vi "PoC writer Eth.vi"() -> ()   [LabVIEW 2022 SP3]
uses:
  JLR/emea-tra-JLR-Synchronization-PoC/PoC_LV2020/Data.ctl
  JLR/emea-tra-JLR-Synchronization-PoC/PoC_LV2020/States.ctl
  <vilib>/xnet/xnet.llb/XNET Frame Ethernet.ctl
  <vilib>/xnet/xnet.llb/XNET Frame Type Ethernet.ctl
  Program Files/National Instruments/LabVIEW 2022/examples/nixnet/projects/NI-XNET Ethernet/subVI/Ethernet/Controls/Ethernet Header.ctl
  Program Files/National Instruments/LabVIEW 2022/examples/nixnet/projects/NI-XNET Ethernet/subVI/Ethernet/Controls/VLAN Tag.ctl
  87a1c0d7-935f-47c0-8fc5-bd666b1ac1f8.vi
  <vilib>/xnet/xnet.llb/XNET Read (State Time Current).vi
  <instrlib>/niSync/niSync.llb/niSync Initialize (Default).vi
  <vilib>/xnet/xnet.llb/XNET Create Session (Frame Output Stream).vi
  <vilib>/xnet/xnet.llb/XNET Write (Frame Ethernet).vi
  <vilib>/xnet/xnet.llb/XNET Read (State Time Trigger).vi
  <resource>/objmgr/xnet.rc
  Program Files/National Instruments/LabVIEW 2022/examples/nixnet/projects/NI-XNET Ethernet/subVI/Ethernet.lvlib
panel:
  out "TimeStamps":timestamp[](array[timestamp]) format="%<%.6X\n%x>T"
  in  "terminal":tag="/Dev2/PFI0"
  in  "terminal 2":tag="/Dev2/PXI_Trig0"
  in  "resource name 2":tag="Dev2"
  in  "Start Time Delay (Seconds)":ext=1.0
  in  "Pulse Width (uS)":ext=1.0
  out "Pulse Start Time":timestamp format="%<%I:%M:%S%6u %p\n%x>T"
  in  "Send Trigger":bool
  out "Time Trigger Received":timestamp caption="network time trigger" format="%<%.6X\n%x>T"
  out "UTC Offset (s)":i32
  out "Port State":u32(ring)=3 items=["Disabled"=3, "Master"=6, "Passive"=7, "Slave"=9]
  out "Time Diff (Sync vs Xnet) (s)":dbl format="%#.6f"
  out "Adj Time Diff (Sync vs Xnet) (s)":dbl format="%#.6f"
  in  "payload 2":string="\u0000\u0001\u0002\u0003\u0004\u0005\u0006\u0007\b\t\n\u000b\f\r\u000e\u000f\u0010\u0011\u0012\u0013\u0014\u0015\u0016\u0017\u0018\u0019\u001a\u001b\u001c\u001d\u001e\u001f !\"#$%&'()*+,-./0123456789:;<=>?@ABCDEFGHIJKLMNOPQRSTUVWXYZ[\\]^_`abc"
  in  "destination MAC address":cluster{u8, u8, u8, u8, u8, u8}={255, 255, 255, 255, 255, 255} {"?" format="%.0x"; "?" format="%.0x"; "?" format="%.0x"; "?" format="%.0x"; "?" format="%.0x"; "?" format="%.0x"}
  in  "Has VLAN Tag":bool=TRUE
  in  "Ethertype":u16=34997 format="%.0x"
  in  "VID":u16=2
  in  "priority":u8=3
  in  "Write Frame":bool
  out "Frames sent":u32
  out "Time elapsed to set OS time (s)":dbl format="%#.6f"
  in  "gPtP master interface":refnum<k21>="ENET1"
  in  "NI Sync Resource Name":tag="Dev2"
  in  "Stop 2":bool
  out "Cluster":T1 {"OS time set at" format="%<%.6X\n%x>T"; "Time Trigger Received" format="%<%.6X\n%x>T"}
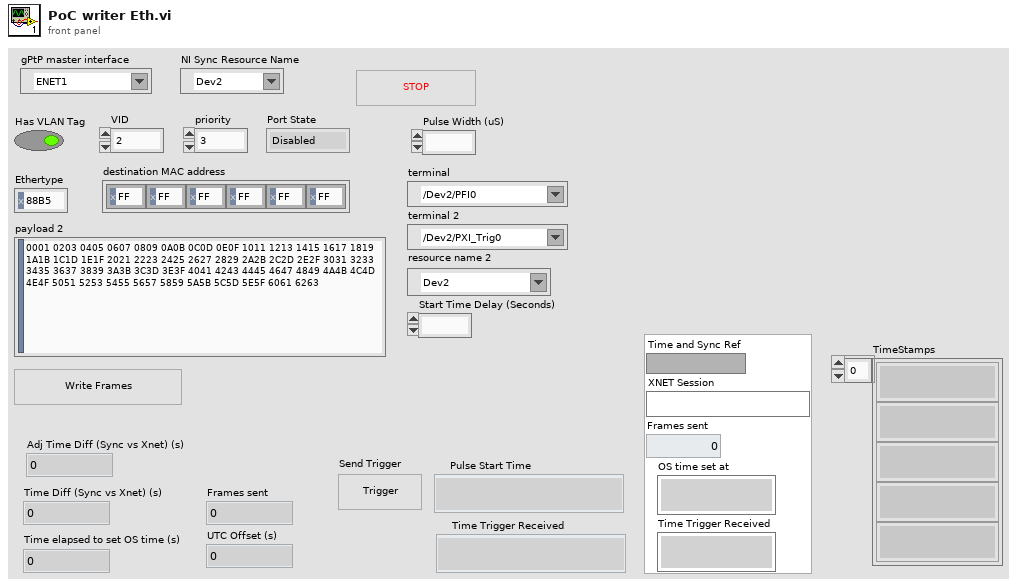
[diagram p1: front panel]
types:
  T1 = typedef "Data.ctl" = cluster{"Time and Sync Ref":refnum<k15>, "XNET Session":refnum<k21>, "Frames sent":u32, "OS time set at":timestamp, "Time Trigger Received":timestamp}
  T2 = enum16{"open", "open or create", "create or replace", "create", "open (read-only)"}
  T3 = typedef "States.ctl" = enum16{"Init 8523", "Init 6683", "Sync 8523", "PPS+Trigger", "Set Sync Time", "Init 8510", "Adjust XNET time", "Idle", "Error"}
  T4 = typedef "States.ctl" = enum16{"Init NI Sync", "Adjust XNET time", "Init XNET", "Update OS time", "Write XNET Frame", "Error", "Idle", "Read Trigger"}
  T5 = typedef "Ethernet.lvlib/VLAN Tag.ctl" = cluster{"TPID":u16, "priority":u8, "DEI":bool, "VID":u16}
  T6 = typedef "Ethernet.lvlib/Ethernet Header.ctl" = cluster{"destination MAC address":cluster{u8, u8, u8, u8, u8, u8}, "source MAC address":cluster{u8, u8, u8, u8, u8, u8}, "Has VLAN Tag":bool, "VLAN Tag":T5, "Ethertype":u16}
  T7 = typedef "XNET Frame Ethernet.ctl" = cluster{"local timestamp":timestamp, "network timestamp":timestamp, "frame data":u8[], "fcs":u32, "type":T8, "network synced?":bool, "receive?":bool, "transmit?":bool, "error?":bool}
  T8 = typedef "XNET Frame Type Ethernet.ctl" = u16
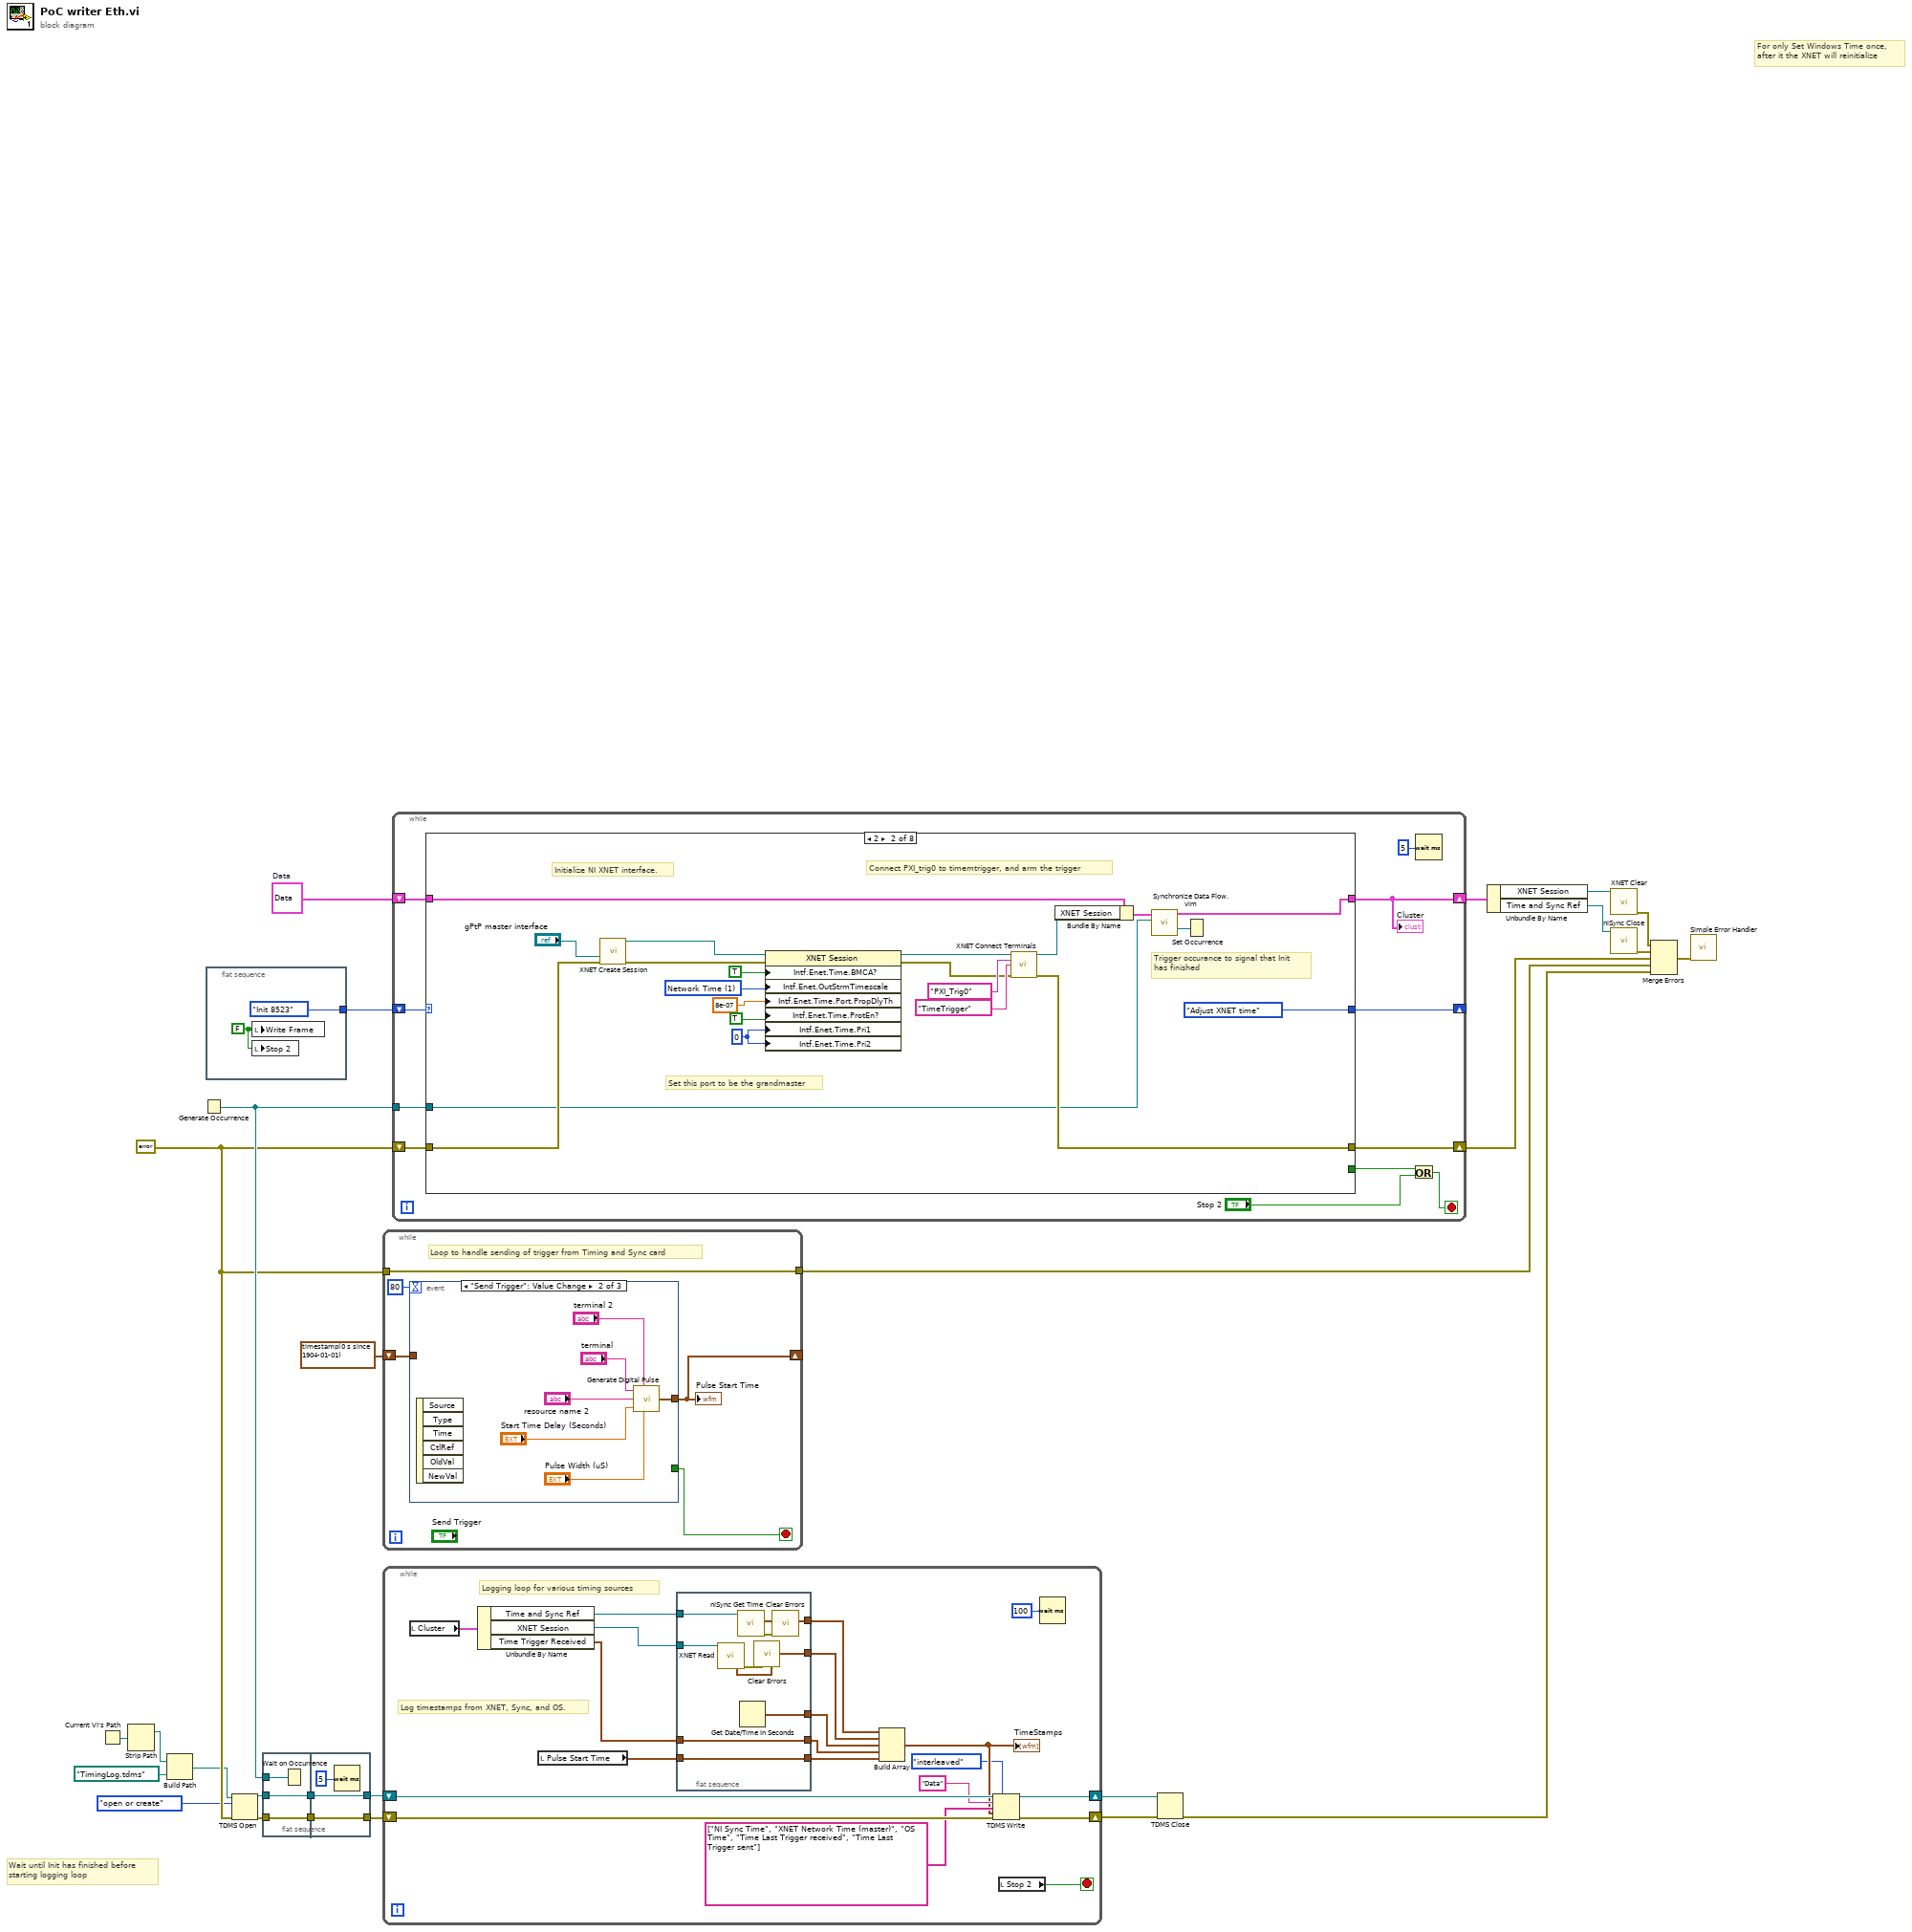
[diagram p0: block diagram]
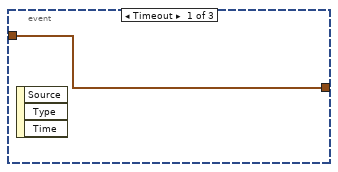
[diagram p2: hidden frame]
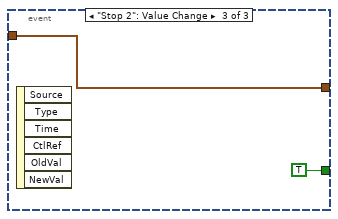
[diagram p3: hidden frame]
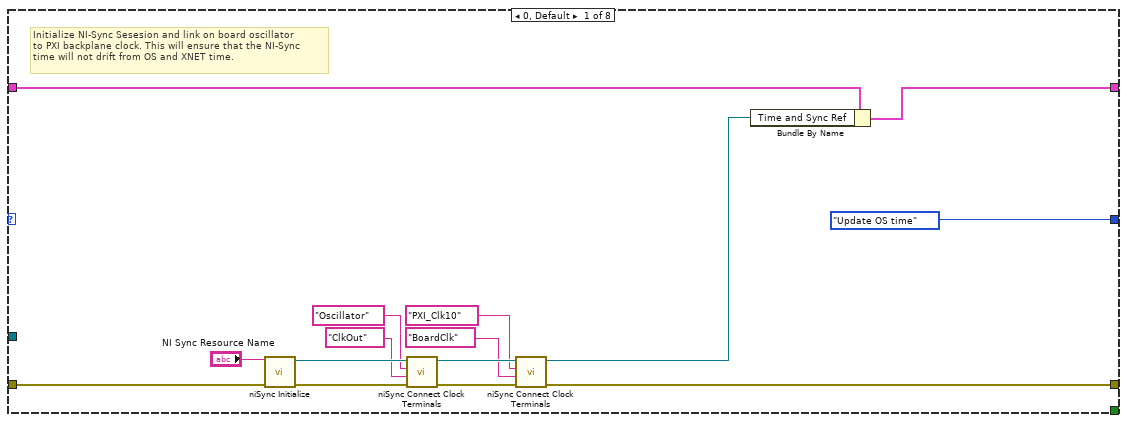
[diagram p4: hidden frame]
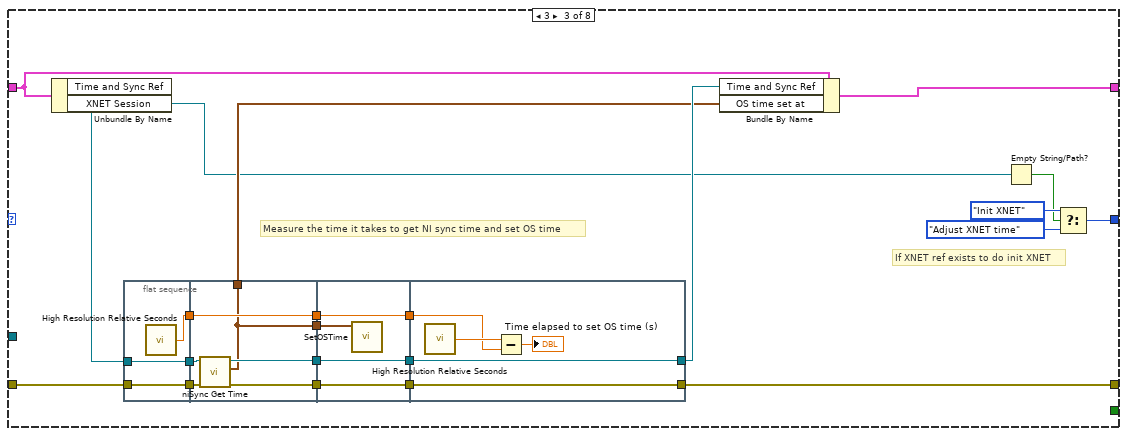
[diagram p5: hidden frame]
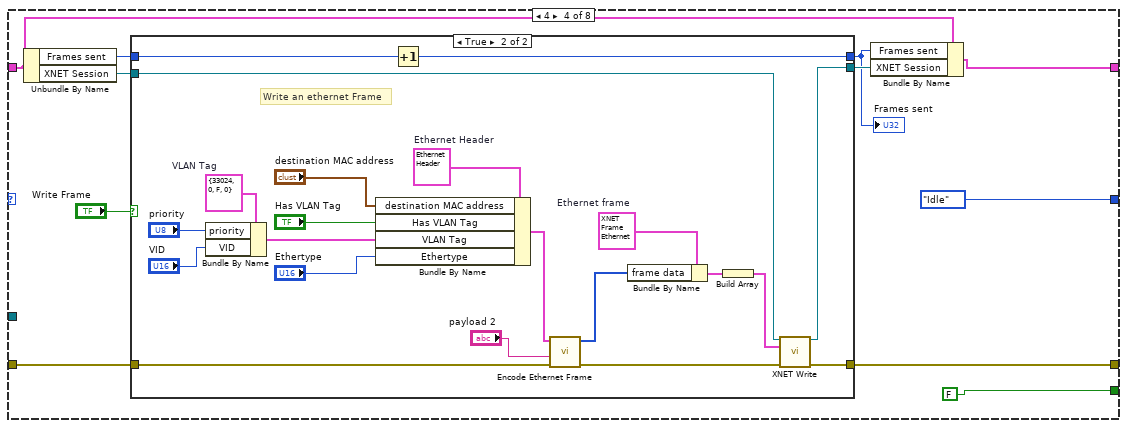
[diagram p6: hidden frame]
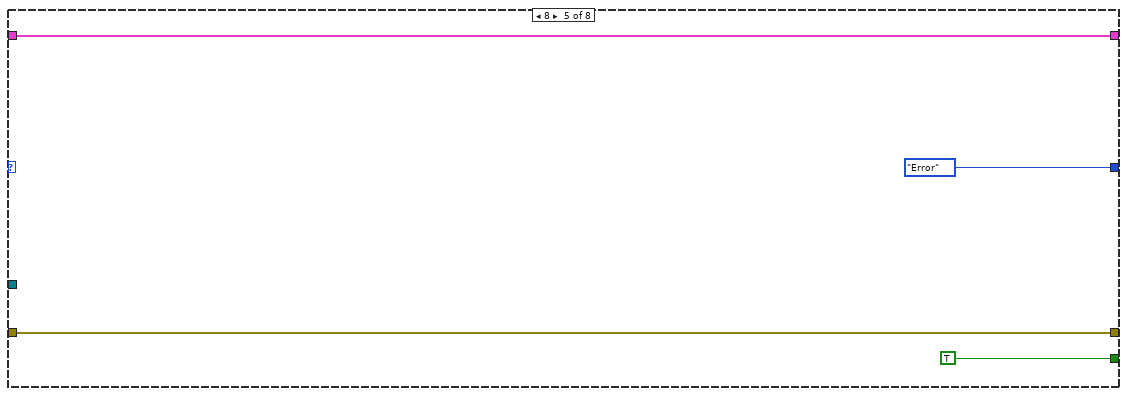
[diagram p8: hidden frame]
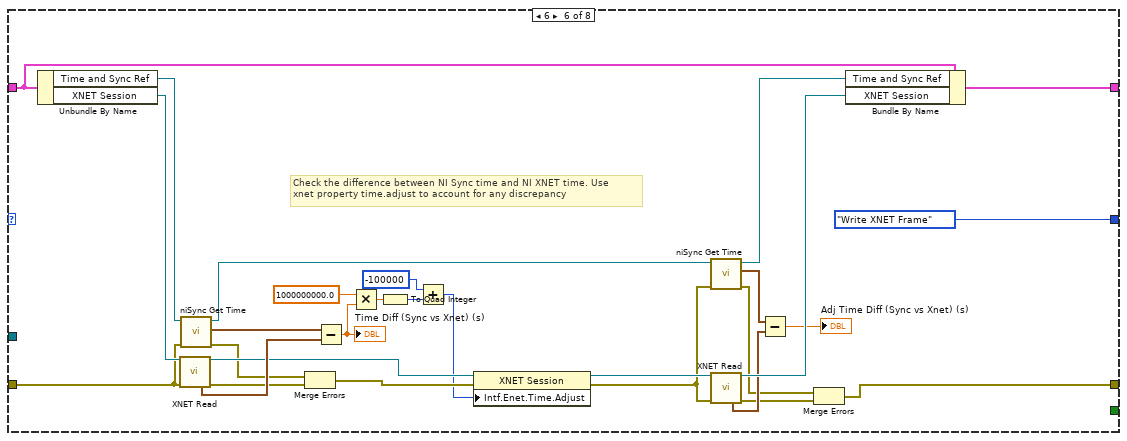
[diagram p9: hidden frame]
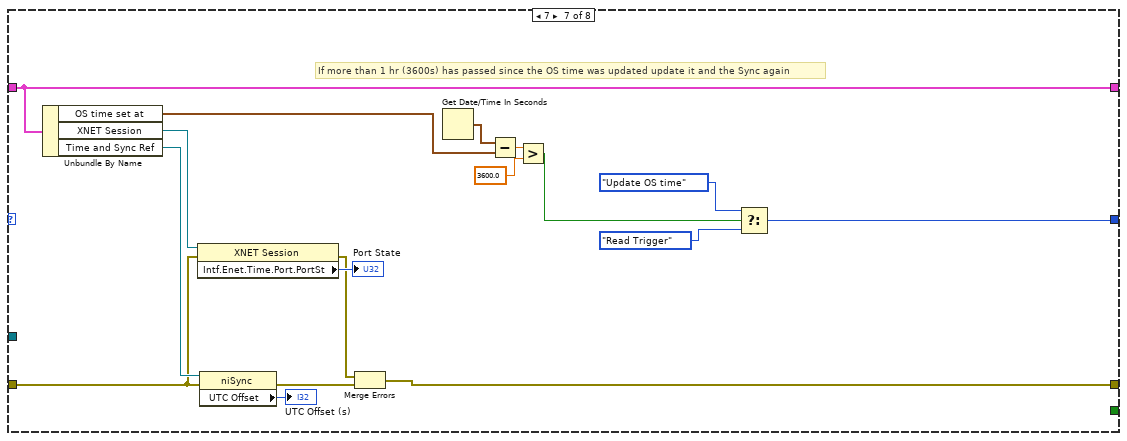
[diagram p10: hidden frame]
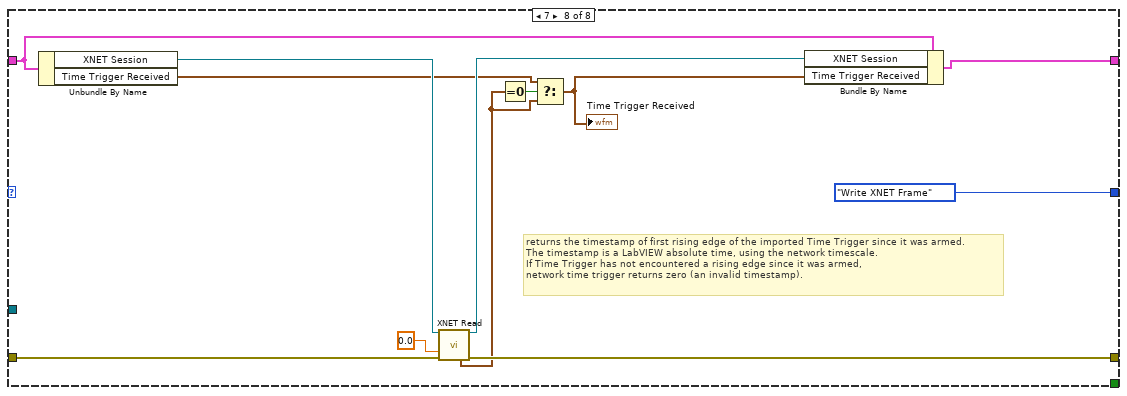
[diagram p11: hidden frame]
diagram:
  w12 = errorcluster {"status"=FALSE, "code"=0, "source"=""} ("error out")
  w24 = T1 {"Time and Sync Ref"="", "XNET Session"="", "Frames sent"=0, "OS time set at"=timestamp(0 s since 1904-01-01), "Time Trigger Received"=timestamp(0 s since 1904-01-01)}  # Data
  # "Wait until Init has finished before \nstarting logging loop"
  # "For only Set Windows Time once,\nafter it the XNET will reinitialize"
  n1 = Current VI's Path() -> (path=w3:path)
  n2 = Strip Path(path=w3) -> (stripped path=w2:path)  [unwired: 1 out]
  n3 = Build Path(base path=w2, name or relative path=path "TimingLog.tdms") -> (appended path=w4:path)
  n4 = Generate Occurrence() -> (w15:refnum<k4>)
  n5 = flat-sequence {
    tunnel: [States."Init 8523"] -> w25
    frame #0 {
      w28 = FALSE ("Write Frame")
      n6 = local write "Write Frame"(w28) -> ()
      n7 = local write "Stop 2"(w28) -> ()
    }
  }
  n8 = TDMS Open(8:w12, 10:T2."open or create" ("operation (0:open)"), 11:w4) -> (0:w9:errorcluster, 3:w11:refnum<k34>)  [unwired: 4 in]
  n9 = flat-sequence {
    tunnel: w15 -> [w32]
    tunnel: w11 -> [w31]
    tunnel: w9 -> [w30]
    tunnel: [w31] -> w27
    tunnel: [w30] -> w26
    tunnel: [w34] -> w8
    tunnel: [w35] -> w10
    tunnel: w27 -> [w35]
    tunnel: w26 -> [w34]
    frame #0 {
      n10 = Wait on Occurrence(2:w32) -> ()  [unwired: 2 in, 1 out]
    }
    frame #1 {
      n11 = Wait (ms)(milliseconds to wait=u32 5) -> ()  [unwired: 1 out]
    }
  }
  n12 = while {
    tunnel: w12 -> [w40]
    tunnel: [w40] -> w16
    shift-right: [w38] -> _
    shift-left: timestamp(0 s since 1904-01-01) ("Pulse Start Time") -> [w37]
    stop <- w39 stop-if-true
    # "Loop to handle sending of trigger from Timing and Sync card"
    n13 = event shown="[1] \"Send Trigger\": Value Change" {
      selector: _ -> [_ _ _]
      dyn-events: _ -> [_ _ _]
      timeout: 80 -> [_ _ _]
      tunnel: [w41 w42 w48] -> w38
      tunnel: [_ _ TRUE] -> w39
      tunnel: w37 -> [w41 _ w48]
      event Timeout {
        n14 = event-data() -> ()  [unwired: 1 in, 3 out]
      }
      event "Send Trigger": Value Change {
        n15 = event-data() -> ()  [unwired: 1 in, 6 out]
        n16 = call "Generate Digital Pulse.vi"("terminal"="terminal", "terminal 2"="terminal 2", "resource name"="resource name 2", "Start Time Delay (Seconds)"="Start Time Delay (Seconds)", "Pulse Width (uS)"="Pulse Width (uS)") -> ("Pulse Start Time"=w42:timestamp)
      }
      event "Stop 2": Value Change {
        n17 = event-data() -> ()  [unwired: 1 in, 6 out]
      }
    }
    "Pulse Start Time" <- w38
  }
  n18 = while {
    shift-right: [w62] -> w14
    shift-left: w8 -> [w64]
    shift-right: [w63] -> w13
    shift-left: w10 -> [w65]
    stop <- w53 stop-if-true
    # "Logging loop for various timing sources"
    # "Log timestamps from XNET, Sync, and OS."
    n19 = local read "Cluster"() -> (w58:T1)
    n20 = Unbundle By Name(w58) -> ("Time and Sync Ref"=w69:refnum<k15>, "XNET Session"=w68:refnum<k21>, "Time Trigger Received"=w67:timestamp)
    n21 = local read "Pulse Start Time"() -> (w66:timestamp)
    n22 = flat-sequence {
      tunnel: w69 -> [w78]
      tunnel: w68 -> [w77]
      tunnel: [w76] -> w50
      tunnel: [w75] -> w51
      tunnel: [w74] -> w52
      tunnel: w67 -> [w73]
      tunnel: [w73] -> w55
      tunnel: w66 -> [w72]
      tunnel: [w72] -> w54
      frame #0 {
        n23 = call-poly <vilib>:"XNET Read.vi"("session in"=w77) -> ("network time current"=w75:timestamp, "error out"=w71:errorcluster)  [unwired: 10 in, 3 out]
        n24 = call <instrlib>:"niSync Get Time.vi"("instrument handle"=w78) -> ("error out"=w70:errorcluster, "time"=w74:timestamp)  [unwired: 6 in, 1 out]
        n25 = Get Date/Time In Seconds() -> (seconds since 1Jan1904=w76:timestamp)
        n26 = call <vilib>:"Clear Errors.vi"("error in (no error)"=w71) -> ()  [unwired: 5 in, 2 out]
        n27 = call <vilib>:"Clear Errors.vi"("error in (no error)"=w70) -> ()  [unwired: 5 in, 2 out]
      }
    }
    n28 = Build Array(w52, w51, w50, w55, w54) -> (w57:timestamp[])
    "TimeStamps" <- w57
    n29 = TDMS Write(0:w65, 1:enum16{"decimated", "interleaved"}."interleaved" ("data layout (0:decimated)"), 5:"Data" ("group name in (Untitled)"), 7:string[] ["NI Sync Time", "XNET Network Time (master)", "OS Time", "Time Last Trigger received", "Time Last Trigger sent"] ("channel name(s) in (Untitled)"), 9:w57, 11:w64) -> (4:w63:refnum<k34>, 15:w62:errorcluster)  [unwired: 2 out]
    n30 = local read "Stop 2"() -> (w53:bool)
    n31 = Wait (ms)(milliseconds to wait=u32 100) -> ()  [unwired: 1 out]
  }
  n32 = while {
    shift-right: [w84] -> _
    shift-left: w25 -> [w88]
    shift-right: [w86] -> w20
    shift-left: w12 -> [w85]
    shift-right: [w79] -> w19
    shift-left: w24 -> [w87]
    tunnel: w15 -> [w80]
    stop <- w82 stop-if-true
    n33 = case shown="2" w88 {
      tunnel: w87 -> [w92 w116 w141 w173 w203 w223 w250 w256]
      tunnel: [w94 w109 w133 w175 w201 w207 w234 w257] -> w86
      tunnel: w85 -> [w93 w117 w146 w176 w201 w221 w238 w258]
      tunnel: [w91 w107 w142 w174 w203 w222 w250 w255] -> w79
      tunnel: [States."Update OS time" States."Adjust XNET time" w129 States."Idle" States."Error" States."Write XNET Frame" w243 States."Write XNET Frame"] -> w84
      tunnel: [_ _ _ FALSE TRUE _ _ _] -> w83
      tunnel: w80 -> [_ w105 _ _ _ _ _ _]
      frame 0, Default {
        # "Initialize NI-Sync Sesesion and link on board oscillator \nto PXI backplane clock. This will ensure that the NI-Sync\ntime will not drift from OS and XNET time."
        n34 = call-poly <instrlib>:"niSync Initialize.vi"("error in (no error)"=w93, "resource name"="NI Sync Resource Name") -> ("error out"=w104:errorcluster, "instrument handle out"=w103:refnum<k15>)  [unwired: 8 in]
        n35 = call <instrlib>:"niSync Connect Clock Terminals.vi"("error in (no error)"=w104, "destination terminal"="ClkOut", "source terminal"="Oscillator", "instrument handle"=w103) -> ("error out"=w101:errorcluster, "instrument handle out"=w102:refnum<k15>)  [unwired: 6 in]
        n36 = call <instrlib>:"niSync Connect Clock Terminals.vi"("error in (no error)"=w101, "destination terminal"="BoardClk", "source terminal"="PXI_Clk10", "instrument handle"=w102) -> ("error out"=w94:errorcluster, "instrument handle out"=w95:refnum<k15>)  [unwired: 6 in]
        n37 = Bundle By Name(cluster=w92, "Time and Sync Ref"=w95) -> (w91:T1)
      }
      frame 2 {
        w118 = u32 1 items=["Local Time", "Network Time"] ("Interface:Ethernet:Output Stream Timescale")
        w119 = u32 0 ("Interface:Ethernet:Time Sync:Priority1")
        # "Trigger occurance to signal that Init\nhas finished"
        # "Set this port to be the grandmaster"
        # "Connect PXI_trig0 to timemtrigger, and arm the trigger"
        # "Initialize NI XNET interface."
        n38 = call-poly <vilib>:"XNET Create Session.vi"("interface"="gPtP master interface", "error in (no error)"=w117) -> ("session out"=w123:refnum<k21>, "error out"=w124:errorcluster)  [unwired: 12 in]
        n39 = property class="XNET Session"(reference=w123, error in=w124, "Intf.Enet.Time.BMCA?"=TRUE ("Interface:Ethernet:Time Sync:Protocol Enabled?"), "Intf.Enet.OutStrmTimescale"=w118, "Intf.Enet.Time.Port.PropDlyTh"=8e-07 ("Propagation Delay Threshold (s)"), "Intf.Enet.Time.ProtEn?"=TRUE ("Interface:Ethernet:Time Sync:Protocol Enabled?"), "Intf.Enet.Time.Pri1"=w119, "Intf.Enet.Time.Pri2"=w119) -> (reference out=w112:refnum<k21>, error out=w111:errorcluster)
        n40 = call <vilib>:"XNET Connect Terminals.vi"("session in"=w112, "source terminal"=tag "PXI_Trig0", "destination terminal"=tag "TimeTrigger", "error in (no error)"=w111) -> ("session out"=w110:refnum<k21>, "error out"=w109:errorcluster)  [unwired: 10 in]
        n41 = Bundle By Name(cluster=w116, "XNET Session"=w110) -> (w108:T1)
        n42 = call "Synchronize Data Flow.vim"("input 2"=w105, "input 1"=w108) -> ("output 2"=w106:refnum<k4>, "output 1"=w107:T1)  [unwired: 2 in, 2 out]
        n43 = Set Occurrence(w106) -> ()
      }
      frame 3 {
        # "If XNET ref exists to do init XNET"
        # "Measure the time it takes to get NI sync time and set OS time"
        n44 = Unbundle By Name(w141) -> ("Time and Sync Ref"=w144:refnum<k15>, "XNET Session"=w127:refnum<k21>)
        n45 = flat-sequence {
          tunnel: [w150] -> w147
          tunnel: w146 -> [w149]
          tunnel: [w149] -> w145
          tunnel: w144 -> [w148]
          tunnel: [w148] -> w143
          tunnel: w147 -> [w154]
          tunnel: w145 -> [w153]
          tunnel: w143 -> [w152]
          tunnel: [w156] -> w140
          tunnel: [w155] -> w139
          tunnel: [w154] -> w138
          tunnel: [w151] -> w131
          tunnel: [w151] -> w134
          tunnel: w140 -> [w160]
          tunnel: w139 -> [w159]
          tunnel: w138 -> [w158]
          tunnel: [w160] -> w137
          tunnel: [w159] -> w136
          tunnel: [w158] -> w135
          tunnel: w134 -> [w157]
          tunnel: [w164] -> w133
          tunnel: [w165] -> w132
          tunnel: w137 -> [w165]
          tunnel: w136 -> [w164]
          tunnel: w135 -> [w161]
          frame #0 {
            n46 = call <vilib>:"High Resolution Relative Seconds.vi"() -> ("relative seconds"=w150:dbl)
          }
          frame #1 {
            n47 = call <instrlib>:"niSync Get Time.vi"("error in (no error)"=w153, "instrument handle"=w152) -> ("error out"=w155:errorcluster, "time"=w151:timestamp, "instrument handle out"=w156:refnum<k15>)  [unwired: 5 in]
          }
          frame #2 {
            n48 = call "SetOSTime.vi"("OS time"=w157) -> ()  [unwired: 10 in, 1 out]
          }
          frame #3 {
            n49 = call <vilib>:"High Resolution Relative Seconds.vi"() -> ("relative seconds"=w162:dbl)
            n50 = Subtract(x=w162, y=w161) -> (x-y=→"Time elapsed to set OS time (s)":dbl)
          }
        }
        n51 = Bundle By Name(cluster=w141, "Time and Sync Ref"=w132, "OS time set at"=w131) -> (w142:T1)
        n52 = Empty String/Path?(string/path=w127) -> (empty?=w126:bool)
        n53 = Select(t=States."Init XNET", s=w126, f=States."Adjust XNET time") -> (s? t:f=w129:u16)
      }
      frame 4 {
        n54 = Unbundle By Name(w173) -> ("Frames sent"=w170:u32, "XNET Session"=w172:refnum<k21>)
        n55 = case shown="True" "Write Frame" {
          tunnel: w176 -> [w179 w185]
          tunnel: [w179 w184] -> w175
          tunnel: w172 -> [w177 w183]
          tunnel: [w177 w182] -> w171
          tunnel: w170 -> [w178 w181]
          tunnel: [w178 w180] -> w169
          frame False {
          }
          frame True {
            w190 = T5 {"TPID"=33024, "priority"=0, "DEI"=FALSE, "VID"=0}  # VLAN Tag
            w191 = T6 {"destination MAC address"={0, 0, 0, 0, 0, 0}, "source MAC address"={0, 0, 0, 0, 0, 0}, "Has VLAN Tag"=FALSE, "VLAN Tag"={"TPID"=33024, "priority"=0, "DEI"=FALSE, "VID"=0}, "Ethertype"=0}  # Ethernet Header
            w195 = T7 {"local timestamp"=timestamp(0 s since 1904-01-01), "network timestamp"=timestamp(0 s since 1904-01-01), "frame data"=[], "fcs"=0, "type"=0, "network synced?"=FALSE, "receive?"=FALSE, "transmit?"=FALSE, "error?"=FALSE}  # Ethernet frame
            # "Write an ethernet Frame"
            n56 = Bundle By Name(cluster=w190, "priority"="priority", "VID"="VID") -> (w189:T5)
            n57 = Bundle By Name(cluster=w191, "destination MAC address"="destination MAC address", "Has VLAN Tag"="Has VLAN Tag", "VLAN Tag"=w189, "Ethertype"="Ethertype") -> (w196:T6)
            n58 = Increment(x=w181) -> (x+1=w180:u32)
            n59 = call "Encode Ethernet Frame.vi"("error in (no error)"=w185, "payload"="payload 2", "Ethernet Header"=w196) -> ("error out"=w186:errorcluster, "frame data"=w194:u8[])  [unwired: 7 in]
            n60 = Bundle By Name(cluster=w195, "frame data"=w194) -> (w193:T7)
            n61 = Build Array(w193) -> (w192:T7[])
            n62 = call-poly <vilib>:"XNET Write.vi"("session in"=w183, "data"=w192, "error in (no error)"=w186) -> ("session out"=w182:refnum<k21>, "error out"=w184:errorcluster)  [unwired: 11 in]
          }
        }
        "Frames sent" <- w169
        n63 = Bundle By Name(cluster=w173, "Frames sent"=w169, "XNET Session"=w171) -> (w174:T1)
      }
      frame 8 {
      }
      frame 6 {
        # "Check the difference between NI Sync time and NI XNET time. Use\nxnet property time.adjust to account for any discrepancy"
        n64 = Unbundle By Name(w223) -> ("Time and Sync Ref"=w224:refnum<k15>, "XNET Session"=w225:refnum<k21>)
        n65 = call-poly <vilib>:"XNET Read.vi"("session in"=w225, "error in (no error)"=w221) -> ("session out"=w227:refnum<k21>, "network time current"=w233:timestamp, "error out"=w226:errorcluster)  [unwired: 9 in, 2 out]
        n66 = call <instrlib>:"niSync Get Time.vi"("error in (no error)"=w221, "instrument handle"=w224) -> ("error out"=w219:errorcluster, "time"=w232:timestamp, "instrument handle out"=w215:refnum<k15>)  [unwired: 5 in]
        n67 = Merge Errors(w219, w226) -> (w220:errorcluster)
        n68 = Subtract(x=w232, y=w233) -> (x-y=w231:dbl)
        "Time Diff (Sync vs Xnet) (s)" <- w231
        n69 = Multiply(x=1000000000.0 ("y"), y=w231) -> (x*y=w229:dbl)
        n70 = To Quad Integer(1:w229) -> (0:w228:i64)
        n71 = Add(x=i64 -100000, y=w228) -> (x+y=w206:i64)
        n72 = property class="XNET Session"(reference=w227, error in=w220, "Intf.Enet.Time.Adjust"=w206) -> (reference out=w217:refnum<k21>, error out=w214:errorcluster)
        n73 = call <instrlib>:"niSync Get Time.vi"("error in (no error)"=w214, "instrument handle"=w215) -> ("error out"=w208:errorcluster, "time"=w212:timestamp, "instrument handle out"=w211:refnum<k15>)  [unwired: 5 in]
        n74 = call-poly <vilib>:"XNET Read.vi"("session in"=w217, "error in (no error)"=w214) -> ("session out"=w216:refnum<k21>, "network time current"=w210:timestamp, "error out"=w209:errorcluster)  [unwired: 9 in, 2 out]
        n75 = Subtract(x=w212, y=w210) -> (x-y=→"Adj Time Diff (Sync vs Xnet) (s)":dbl)
        n76 = Merge Errors(w208, w209) -> (w207:errorcluster)
        n77 = Bundle By Name(cluster=w223, "Time and Sync Ref"=w211, "XNET Session"=w216) -> (w222:T1)
      }
      frame 7 {
        # "If more than 1 hr (3600s) has passed since the OS time was updated update it and the Sync again"
        n78 = Unbundle By Name(w250) -> ("OS time set at"=w248:timestamp, "XNET Session"=w239:refnum<k21>, "Time and Sync Ref"=w240:refnum<k15>)
        n79 = property class="XNET Session"(reference=w239, error in=w238) -> (error out=w236:errorcluster, "Intf.Enet.Time.Port.PortSt"=→"Port State":u32)  [unwired: 1 out]
        n80 = property class="niSync"(reference=w240, error in=w238) -> (error out=w235:errorcluster, "UTC Offset"=→"UTC Offset (s)":i32)  [unwired: 1 out]
        n81 = Merge Errors(w236, w235) -> (w234:errorcluster)
        n82 = Get Date/Time In Seconds() -> (seconds since 1Jan1904=w249:timestamp)
        n83 = Subtract(x=w249, y=w248) -> (x-y=w246:dbl)
        n84 = Greater?(x=w246, y=3600.0) -> (0:w244:bool)
        n85 = Select(t=States."Update OS time", s=w244, f=States."Read Trigger") -> (s? t:f=w243:T4)
      }
      frame 7 {
        # "returns the timestamp of first rising edge of the imported Time Trigger since it was armed. \nThe timestamp is a LabVIEW absolute time, using the network timescale. \nIf Time Trigger has not encountered a rising edge since it was armed, \nnetwork time trigger returns zero (an invalid timestamp)."
        n86 = Unbundle By Name(w256) -> ("XNET Session"=w260:refnum<k21>, "Time Trigger Received"=w253:timestamp)
        n87 = call-poly <vilib>:"XNET Read.vi"("session in"=w260, "timeout (10)"=0.0, "error in (no error)"=w258) -> ("session out"=w259:refnum<k21>, "network time trigger"=w252:timestamp, "error out"=w257:errorcluster)  [unwired: 8 in, 2 out]
        n88 = Equal To 0?(x=w252) -> (x = 0?=w254:bool)
        n89 = Select(t=w253, s=w254, f=w252) -> (s? t:f=w251:timestamp)
        "Time Trigger Received" <- w251
        n90 = Bundle By Name(cluster=w256, "XNET Session"=w259, "Time Trigger Received"=w251) -> (w255:T1)
      }
    }
    "Cluster" <- w79
    n91 = Or(x=w83, y="Stop 2") -> (x .or. y?=w82:bool)
    n92 = Wait (ms)(milliseconds to wait=u32 5) -> ()  [unwired: 1 out]
  }
  n93 = TDMS Close(8:w14, 11:w13) -> (0:w6:errorcluster)  [unwired: 1 out]
  n94 = Unbundle By Name(w19) -> ("XNET Session"=w18:refnum<k21>, "Time and Sync Ref"=w17:refnum<k15>)
  n95 = call <vilib>:"XNET Clear.vi"("session in"=w18) -> ("error out"=w23:errorcluster)  [unwired: 14 in]
  n96 = call <instrlib>:"niSync Close.vi"("instrument handle"=w17) -> ("error out"=w21:errorcluster)  [unwired: 10 in]
  n97 = Merge Errors(w23, w21, w20, w16, w6) -> (w22:errorcluster)
  n98 = call <vilib>:"Simple Error Handler.vi"("error in (no error)"=w22) -> ()  [unwired: 4 in, 5 out]
